vi "CloseAllStages.vi"(8 "error in (no error)":errorcluster, 11 "Config In":T1) -> (0 "error out":errorcluster, 3 "Config Out":T1)   [LabVIEW 2019]
uses:
  Settings/Settings.ctl
  Support/Hardware Configuration.ctl
  Support/Camera Configuration.ctl
  E:/DevHardSoftware/MMicroscopy/HardwareAdapter/Camera/Dependencies/PVCamNET.dll
  Camera/Dependencies/PVCamNET.dll
  <vilib>/userdefined/High Color/IMAQdx.ctl
  Logging/Logging Configuration.ctl
  controls/UI Configuration.ctl
  Dependencies/Madlib.dll
  Dependencies/MicroDrive.dll
  Dependencies/TIRF-Lock.dll
  Logging/Logging.lvlib
  Settings/Settings.lvlib
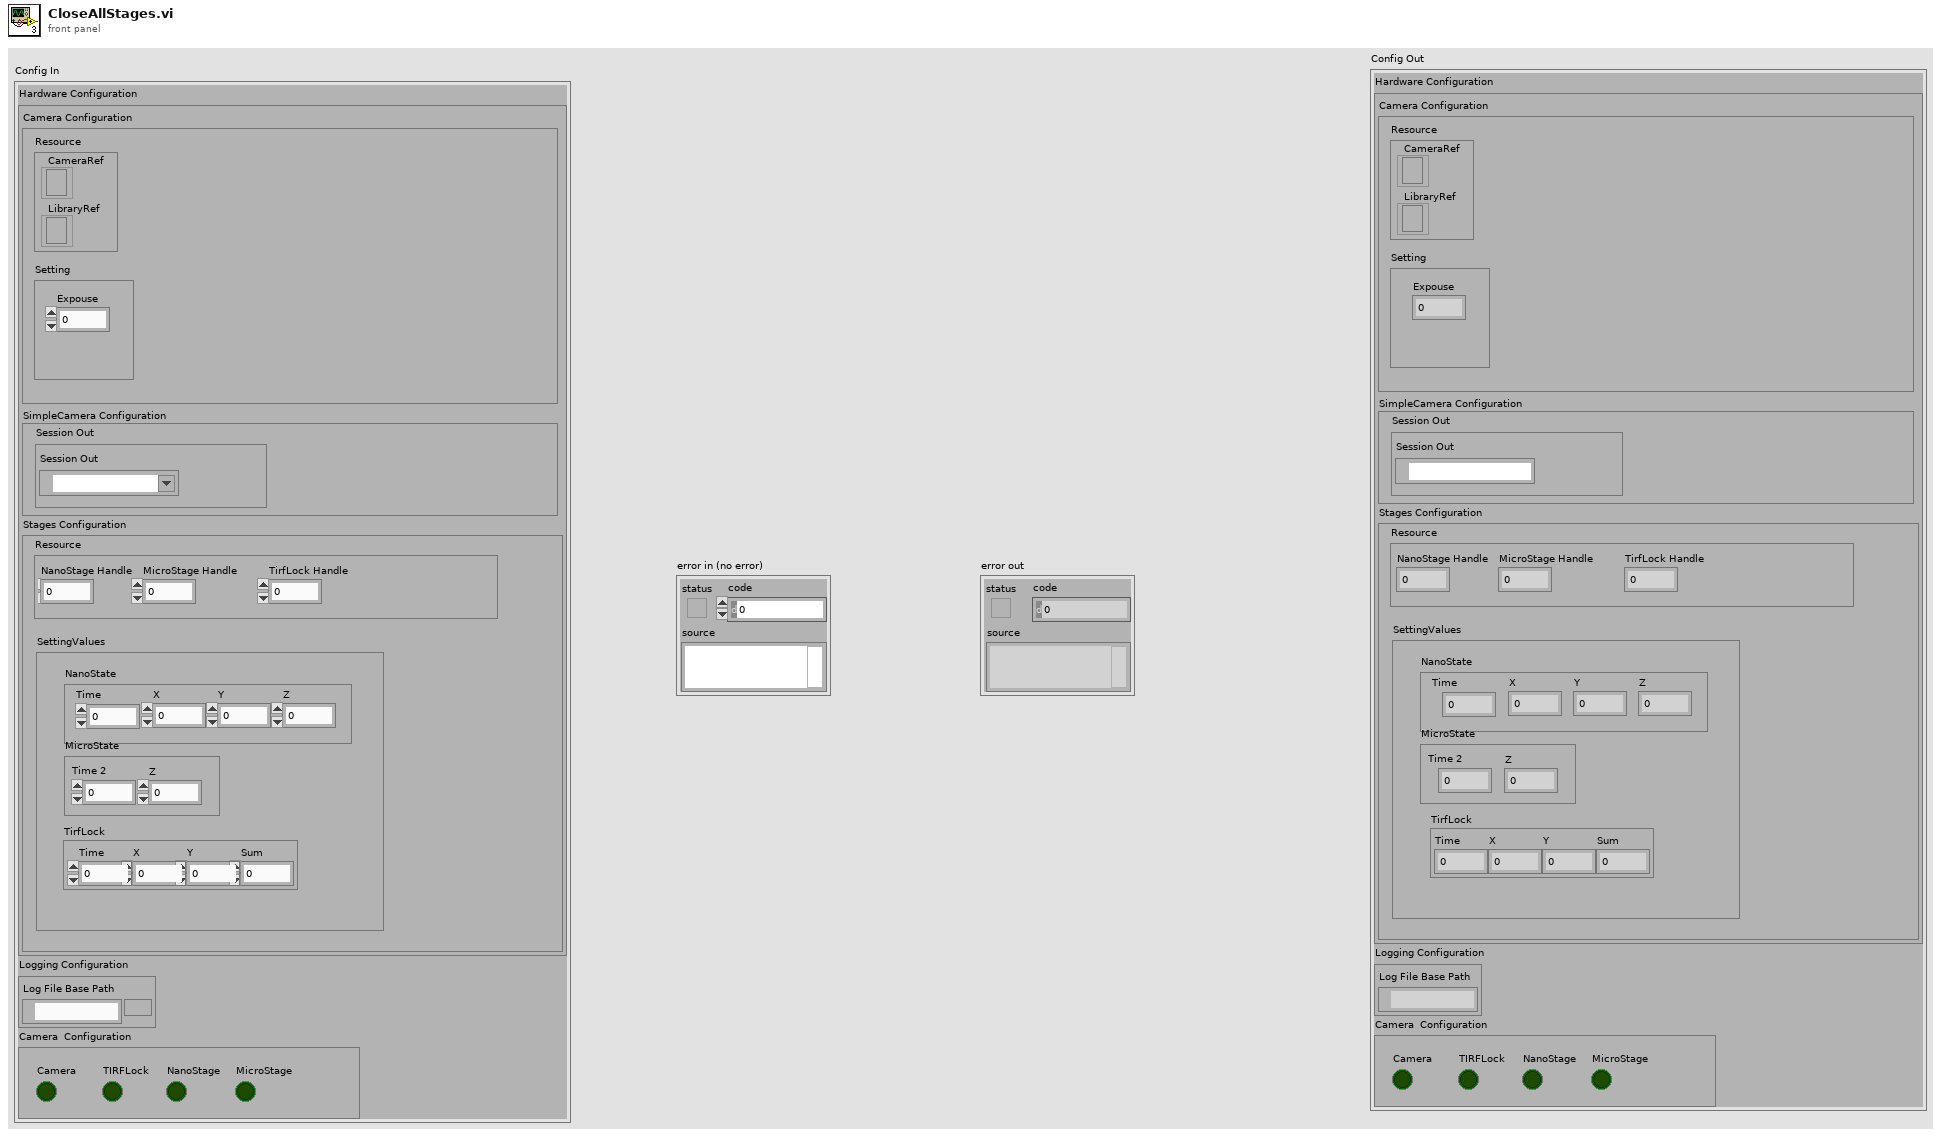
[diagram p1: front panel]
types:
  T1 = typedef "Settings.lvlib/Settings.ctl" = cluster{"Hardware Configuration":T2, "Logging Configuration":T5, "UI Configuration":T6}
  T2 = typedef "Hardware Configuration.ctl" = cluster{"Camera Configuration":T3, "SimpleCamera Configuration":cluster{"Resource":cluster{"Session Out":T4}}, "Stages Configuration":cluster{"Resource":cluster{"NanoStage Handle":i32, "MicroStage Handle":i32, "TirfLock Handle":i32}, "SettingValues":cluster{"NanoState":cluster{"Time":dbl, "X":dbl, "Y":dbl, "Z":dbl}, "MicroState":cluster{"Time 2":dbl, "Z":dbl}, "TirfLock":cluster{"Time":dbl, "X":dbl, "Y":dbl, "Sum":dbl}}}}
  T3 = typedef "Camera Configuration.ctl" = cluster{"Resource":cluster{"CameraRef":refnum<k24>, "LibraryRef":refnum<k24>}, "Setting":cluster{"Expouse":dbl}}
  T4 = typedef "IMAQdx.ctl" = refnum<k21>
  T5 = typedef "Logging.lvlib/Logging Configuration.ctl" = cluster{"Log File Base Path":path}
  T6 = typedef "UI Configuration.ctl" = cluster{"Camera":bool, "NanoStage":bool, "MicroStage":bool, "TIRFLock":bool}
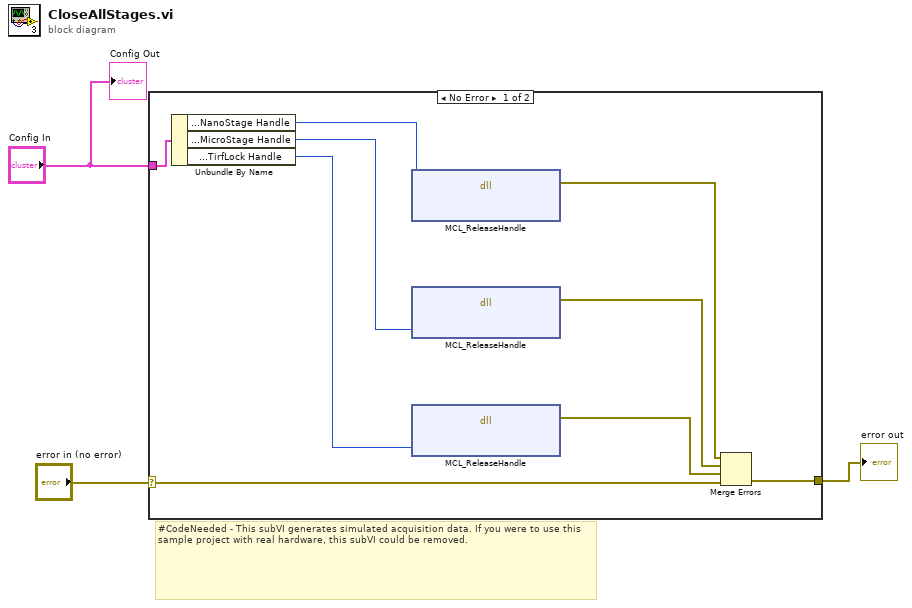
[diagram p0: block diagram]
diagram:
  # "#CodeNeeded - This subVI generates simulated acquisition data. If you were to use this sample project with real hardware, this subVI could be removed."
  n1 = case shown="No Error" "error in (no error)" {
    selector: "error in (no error)" -> [w7 w13]
    tunnel: [w8 w13] -> w2
    tunnel: "Config In" -> [w12 _]
    frame No Error {
      n2 = Unbundle By Name(w12) -> ("Hardware Configuration.Stages Configuration.Resource.NanoStage Handle"=w11:i32, "Hardware Configuration.Stages Configuration.Resource.MicroStage Handle"=w10:i32, "Hardware Configuration.Stages Configuration.Resource.TirfLock Handle"=w9:i32)
      n3 = dll-call lib="E:/DevHardSoftware/MMicroscopy/HardwareAdapter/Stages/Dependencies/Madlib.dll" fn="MCL_ReleaseHandle"("handle"=w11) -> (error out=w4:errorcluster)  [unwired: 4 in, 2 out]
      n4 = dll-call lib="E:/DevHardSoftware/MMicroscopy/HardwareAdapter/Stages/Dependencies/MicroDrive.dll" fn="MCL_ReleaseHandle"("handle"=w10) -> (error out=w5:errorcluster)  [unwired: 4 in, 2 out]
      n5 = dll-call lib="E:/DevHardSoftware/MMicroscopy/HardwareAdapter/Stages/Dependencies/TIRF-Lock.dll" fn="MCL_ReleaseHandle"("handle"=w9) -> (error out=w6:errorcluster)  [unwired: 4 in, 2 out]
      n6 = Merge Errors(w4, w5, w6, w7) -> (w8:errorcluster)
    }
    frame Error {
    }
  }
  "error out" <- w2
  "Config Out" <- "Config In"
